vi "Parameter_check.vi"(6 "Machine_Number":string, 7 "reference":refnum<vi>, 8 "error in":errorcluster, 9 "index":i32, 10 "ACTUAL  PLC PRODUCT CODE":i32, 11 "Cluster":T2={"Product List"=[], "SQL reference"=refnum, "Indicator refrence"=[], "Station Number"=[], "Shift Time stamp"=[timestamp(3597615000 s since 1904-01-01), timestamp(3597658199 s since 1904-01-01), timestamp(3597658200 s since 1904-01-01), timestamp(3597614999 s since 1904-01-01), timestamp(3597589800 s since 1904-01-01), timestamp(3597589800 s since 1904-01-01)], "Com Status Station"=[], "ALARAM INDICATOR REF"=[], "Reading"=[], "Read Parameteres"=[], "Station Name"=[], "Oven Read Parameteres"=[]} {"Shift Time stamp" format="%<%X>T"}) -> (0 "error out":errorcluster, 3 "out of range ?":bool)   [LabVIEW 2017]
uses:
  Controls/station_wise_loop_data.ctl
  <vilib>/addons/database/Connection.llb/Conn ObjectReference.ctl
  <vilib>/addons/database/NI_Database_API.lvlib
panel:
  out "MR_RETURN_TIME":dbl format="%#_g Sec"
  out "1":T1 caption="150T-1" {"PRESSURE_2nd" format="%#_g bar"; "PRESSURE_1st" format="%#_g bar"; "HOLDING_TIME" format="%#_g Sec"; "MR_RETURN_TIME" format="%#_g Sec"}
  out "Read Parameteres 3":string[][](array[string])
  out "Read Parameteres":string[][](array[string])
  out "Machine para Indicator":bool
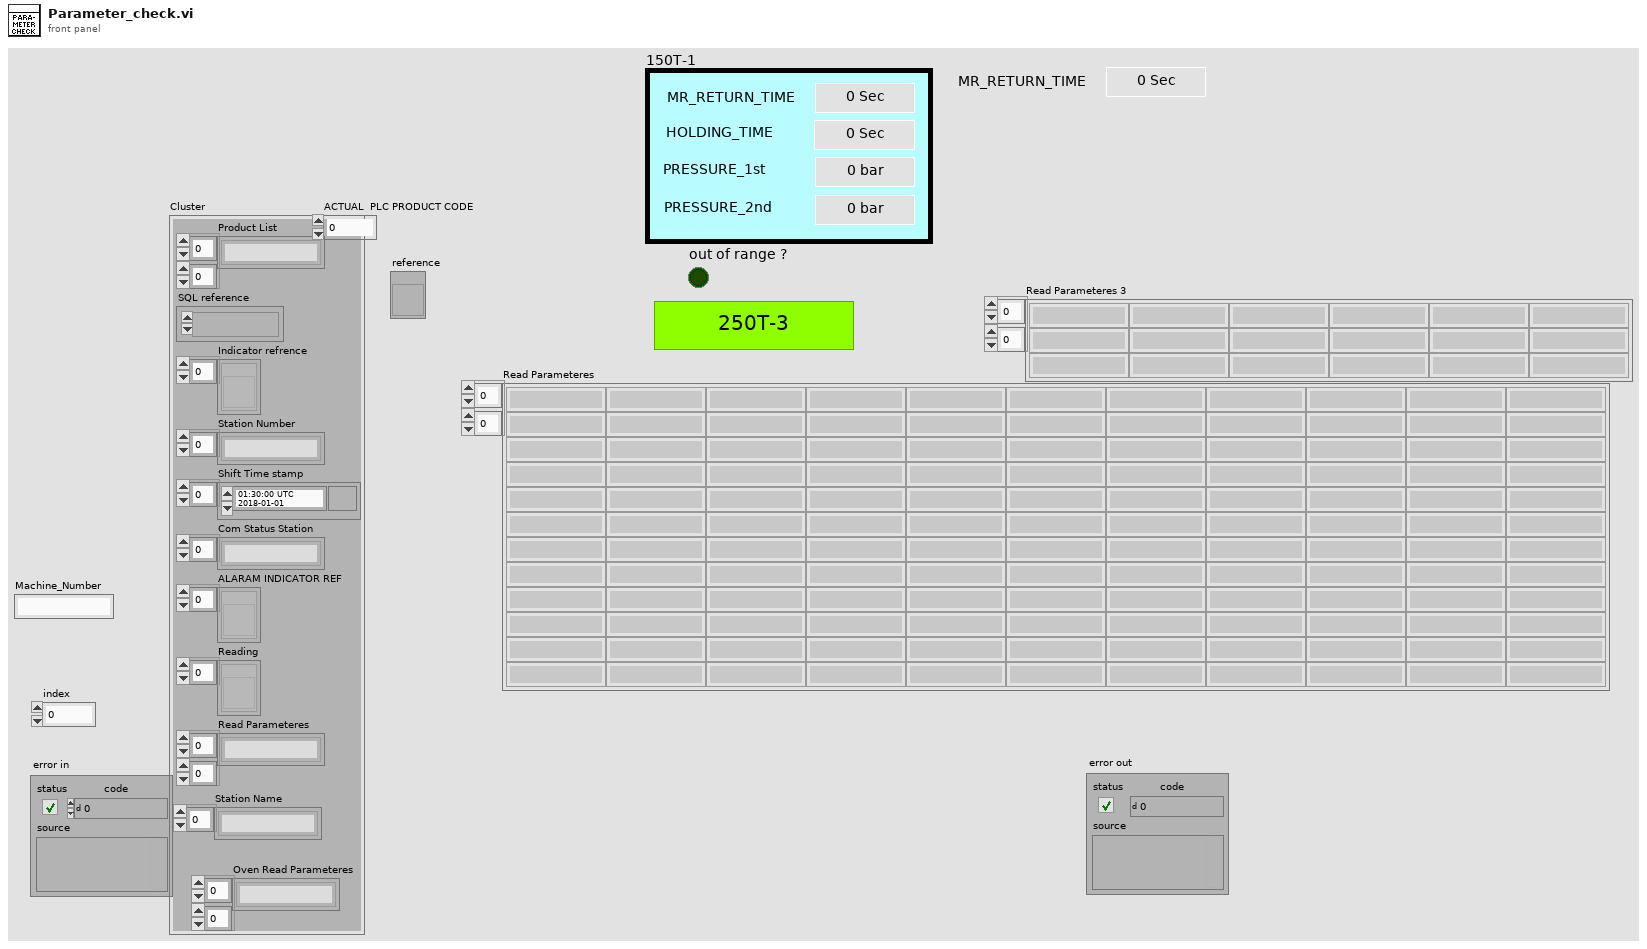
[diagram p1: front panel]
types:
  T1 = cluster{"MR_RETURN_TIME":dbl, "HOLDING_TIME":dbl, "PRESSURE_1st":dbl, "PRESSURE_2nd":dbl}
  T2 = typedef "station_wise_loop_data.ctl" = cluster{"Product List":string[][], "SQL reference":T3, "Indicator refrence":refnum<vi>[], "Station Number":string[], "Shift Time stamp":timestamp[], "Com Status Station":string[], "ALARAM INDICATOR REF":refnum<vi>[], "Reading":refnum<vi>[], "Read Parameteres":string[][], "Station Name":string[], "Oven Read Parameteres":string[][]}
  T3 = typedef "NI_Database_API.lvlib/Conn ObjectReference.ctl" = refnum<k1>
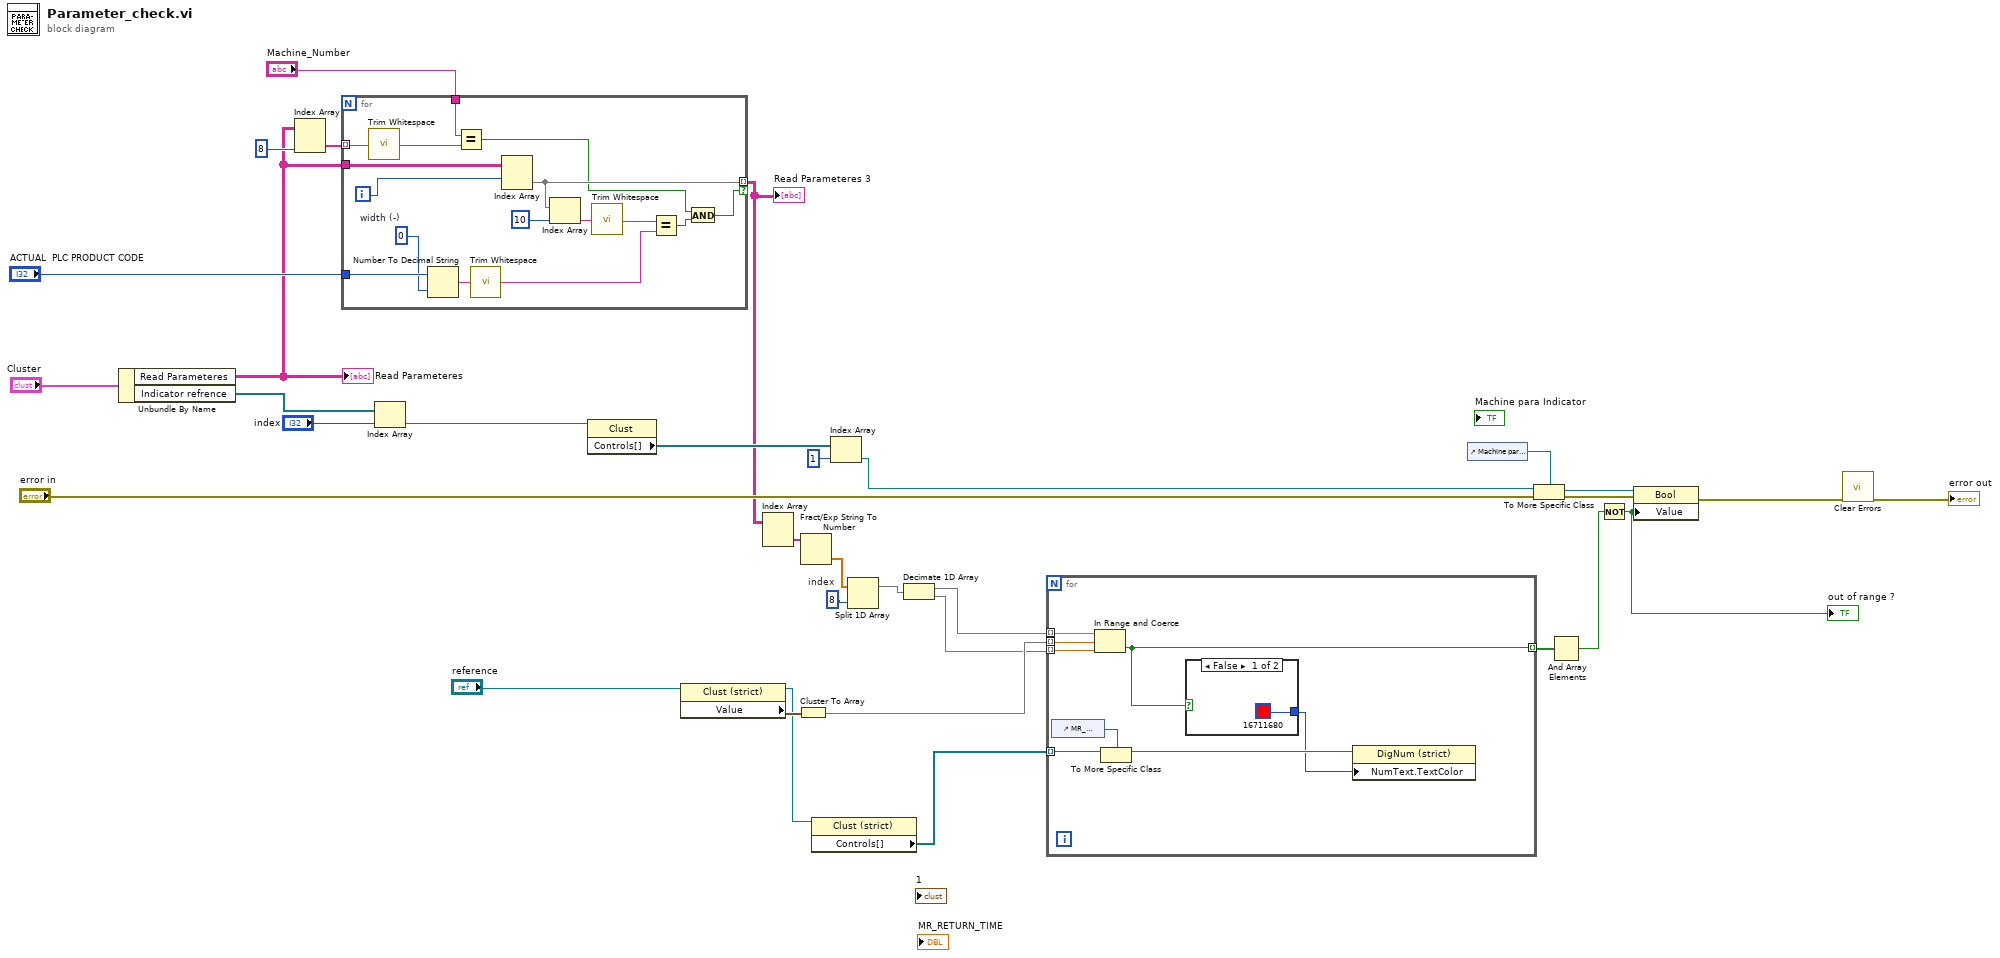
[diagram p0: block diagram]
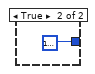
[diagram p2: hidden frame]
diagram:
  w6 = 8  # index
  n1 = Unbundle By Name("Cluster") -> ("Read Parameteres"=w10:string[][], "Indicator refrence"=w28:refnum<vi>[])
  "Read Parameteres" <- w10
  n2 = Index Array(array=w10, index (col)=8 ("disabled index (col)")) -> (element=w30:string[])  [unwired: 1 in]
  n3 = for {
    tunnel: w30 -> [w49] mode=indexing
    tunnel: "Machine_Number" -> [w47]
    tunnel: w10 -> [w45]
    tunnel: [w44] -> w14 mode=indexing if=w38
    tunnel: "ACTUAL  PLC PRODUCT CODE" -> [w37]
    i -> [w46]
    w34 = i16 0  # width (-)
    n4 = call <vilib>:"Trim Whitespace.vi"("string"=w49) -> ("trimmed string"=w48:string)  [unwired: 1 in]
    n5 = Number To Decimal String(number=w37, width (-)=w34) -> (decimal integer string=w36:string)
    n6 = Equal?(x=w47, y=w48) -> (x = y?=w39:bool)
    n7 = call <vilib>:"Trim Whitespace.vi"("string"=w36) -> ("trimmed string"=w35:string)  [unwired: 1 in]
    n8 = Index Array(array=w45, index (row)=w46) -> (element=w44:string[])  [unwired: 1 in]
    n9 = Index Array(array=w44, index=10) -> (element=w42:string)
    n10 = call <vilib>:"Trim Whitespace.vi"("string"=w42) -> ("trimmed string"=w41:string)  [unwired: 1 in]
    n11 = Equal?(x=w41, y=w35) -> (x = y?=w40:bool)
    n12 = And(x=w39, y=w40) -> (x .and. y?=w38:bool)
  }
  "Read Parameteres 3" <- w14
  n13 = Index Array(array=w28, index="index") -> (element=w26:refnum<vi>)
  n14 = property on="Property Node" class="Clust"(reference=w26) -> ("Controls[]"=w25:refnum<vi>[])  [unwired: 1 in, 2 out]
  n15 = property on="Property Node" class="Clust (strict)"(reference="reference") -> (reference out=w7:refnum<vi>, "Value"=w11:T1)  [unwired: 1 in, 1 out]
  n16 = Index Array(array=w14) -> (element=w13:string[])  [unwired: 2 in]
  n17 = Cluster To Array(cluster=w11) -> (array=w2:dbl[])
  n18 = Fract/Exp String To Number(string=w13) -> (number=w5:dbl[])  [unwired: 3 in, 1 out]
  n19 = property on="Property Node" class="Clust (strict)"(reference=w7) -> ("Controls[]"=w8:refnum<vi>[])  [unwired: 1 in, 2 out]
  n20 = Index Array(array=w25, index=1) -> (element=w22:refnum<vi>)
  n21 = Split 1D Array(array=w5, index=w6) -> (first subarray=w4:dbl[])  [unwired: 1 out]
  n22 = Decimate 1D Array(w4) -> (w3:dbl[], w1:dbl[])
  n23 = for {
    tunnel: [w54] -> w12 mode=indexing
    tunnel: w3 -> [w57] mode=indexing
    tunnel: w1 -> [w56] mode=indexing
    tunnel: w2 -> [w55] mode=indexing
    tunnel: w8 -> [w53] mode=indexing
    n24 = control-ref of="MR_RETURN_TIME"() -> (w52:refnum<vi>)
    n25 = In Range and Coerce(upper limit=w57, x=w55, lower limit=w56) -> (In Range?=w54:bool)  [unwired: 1 out]
    n26 = To More Specific Class(target class=w52, reference=w53) -> (specific class reference=w51:refnum<vi>)  [unwired: 1 in, 1 out]
    n27 = case shown="False" w54 {
      tunnel: [u32 16711680 ("Numeric Text.Text Colors:BG Color 2") u32 16777222 ("Numeric Text.Text Colors:BG Color 2")] -> w50
      frame False {
      }
      frame True {
      }
    }
    n28 = property on="Property Node" class="DigNum (strict)"(reference=w51, "NumText.TextColor"=w50) -> ()  [unwired: 1 in, 2 out]
  }
  n29 = control-ref of="Machine para Indicator"() -> (w21:refnum<vi>)
  n30 = To More Specific Class(target class=w21, reference=w22, error in="error in") -> (specific class reference=w20:refnum<vi>, error out=w23:errorcluster)
  n31 = And Array Elements(Boolean array=w12) -> (logical AND=w17:bool)
  n32 = Not(x=w17) -> (.not. x?=w18:bool)
  "out of range ?" <- w18
  n33 = property on="Property Node" class="Bool"(reference=w20, error in=w23, "Value"=w18) -> (error out=w19:errorcluster)  [unwired: 1 out]
  n34 = call <vilib>:"Clear Errors.vi"("error in (no error)"=w19) -> ("error out"=→"error out":errorcluster)  [unwired: 5 in, 1 out]
